vi "Read.vi"(8 "error in (no error)":errorcluster, 9 "Variant":variant, 11 "RS232 in":refnum<class "RS-xxx.lvclass">) -> (0 "error out":errorcluster, 2 "String":string, 3 "RS232 out":refnum<class "RS-xxx.lvclass">)   [LabVIEW 2013, in "Protocol Classes.lvlib" / "RS-xxx.lvclass"]
uses:
  RS-xxx.lvclass
  Protocol Parent/Methods/Read Parameter.ctl
  RS-xxx.lvclass/RS-xxx.ctl
  Data Access/Read Port Ref.vi
  Data Access/Read PortSettings.vi
  Data Access/Write Port Ref.vi
  Protocol Parent/Protocol Parent.lvclass
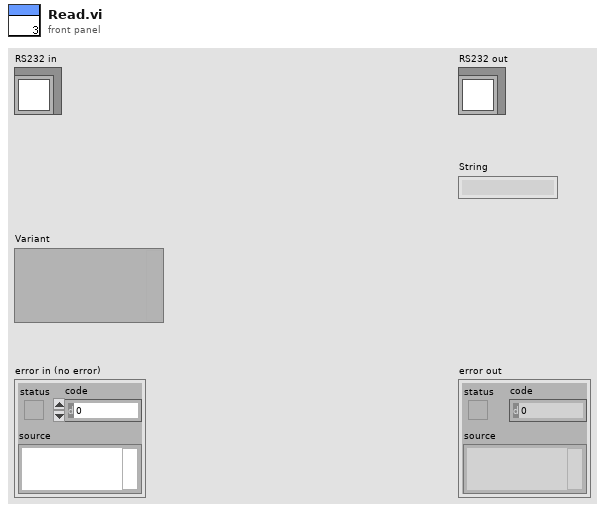
[diagram p1: front panel]
types:
  T1 = typedef "Protocol Classes.lvlib/Protocol Parent.lvclass/Read Parameter.ctl" = cluster{"Wait Type":enum16{"Byte Count", "Wait sec"}, "Wait Value":dbl}
  T2 = cluster{"Port":string, "Baud Rate":u32, "Data Bits":u16, "Parity":enum16{"None", "Odd", "Even", "Mark", "Space"}, "Stop Bits":u16, "Flow Control":u16, "XON":enum16{"NUL", "SOH", "STX", "ETX", "EOT", "ENQ", "ACK", "BEL", "BS", "HT", "LF", "VT", "FF", "CR", "SO", "SI", "DLE", "DC1", "DC2", "DC3", "DC4", "NAK", "SYN", "ETB", "CAN", "EM", "SUB", "ESC", "FS", "GS", "RS", "US", "SP", "!", "\"", "#", "$", "%", "&", "'", "(", ")", "*", "+", ",", "- (-)", ".", "/", "0", "1", "2", "3", "4", "5", "6", "7", "8", "9", ":", ";", "<", "=", ">", "?", "@", "A", "B", "C", "D", "E", "F", "G", "H", "I", "J", "K", "L", "M", "N", "O", "P", "Q", "R", "S", "T", "U", "V", "W", "X", "Y", "Z", "[", "\\", "]", "^", "_", "`", "a", "b", "c", "d", "e", "f", "g", "h", "i", "j", "k", "l", "m", "n", "o", "p", "q", "r", "s", "t", "u", "v", "w", "x", "y", "z", "{", "|", "}", "~"}, "XOFF":enum16{"NUL", "SOH", "STX", "ETX", "EOT", "ENQ", "ACK", "BEL", "BS", "HT", "LF", "VT", "FF", "CR", "SO", "SI", "DLE", "DC1", "DC2", "DC3", "DC4", "NAK", "SYN", "ETB", "CAN", "EM", "SUB", "ESC", "FS", "GS", "RS", "US", "SP", "!", "\"", "#", "$", "%", "&", "'", "(", ")", "*", "+", ",", "- (-)", ".", "/", "0", "1", "2", "3", "4", "5", "6", "7", "8", "9", ":", ";", "<", "=", ">", "?", "@", "A", "B", "C", "D", "E", "F", "G", "H", "I", "J", "K", "L", "M", "N", "O", "P", "Q", "R", "S", "T", "U", "V", "W", "X", "Y", "Z", "[", "\\", "]", "^", "_", "`", "a", "b", "c", "d", "e", "f", "g", "h", "i", "j", "k", "l", "m", "n", "o", "p", "q", "r", "s", "t", "u", "v", "w", "x", "y", "z", "{", "|", "}", "~"}, "End Read on Termination Character":bool, "End Write on Termination Character":bool, "Termination Character":u8}
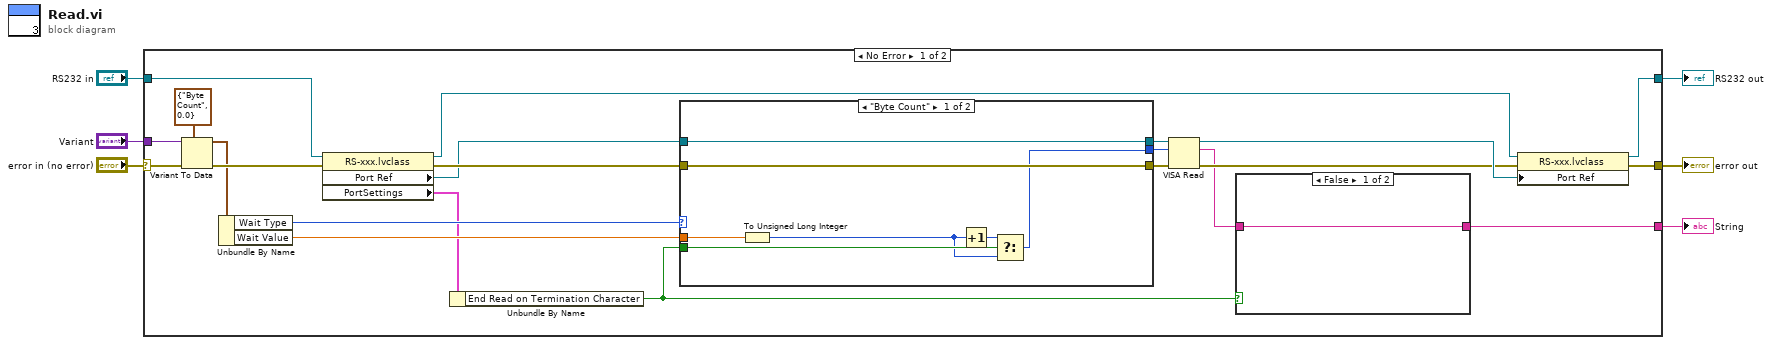
[diagram p0: block diagram]
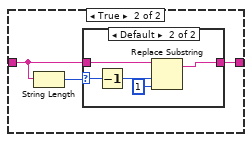
[diagram p2: hidden frame]
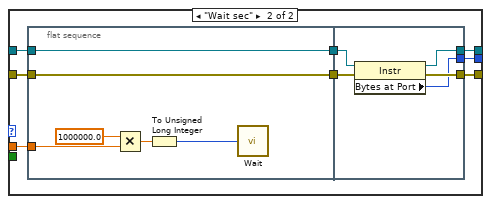
[diagram p4: hidden frame]
diagram:
  n1 = case shown="No Error" "error in (no error)" {
    selector: "error in (no error)" -> [w22 w66]
    tunnel: "RS232 in" -> [w28 w65]
    tunnel: [w25 w66] -> w2
    tunnel: [w23 w65] -> w4
    tunnel: "Variant" -> [w20 _]
    tunnel: [w8 _] -> w1
    frame No Error {
      n2 = Variant To Data(error in=w22, type=T1 {"Wait Type"=enum."Byte Count", "Wait Value"=0.0} ("Read Parameter"), Variant=w20) -> (data=w19:T1, error out=w21:errorcluster)
      n3 = Unbundle By Name(w19) -> ("Wait Type"=w13:enum16{"Byte Count", "Wait sec"}, "Wait Value"=w12:dbl)
      n4 = property class="RS-xxx.lvclass"(reference=w28, error in=w21) -> (reference out=w24:refnum<class "RS-xxx.lvclass">, error out=w18:errorcluster, "Port Ref"=w17:refnum<visa-resource-name>, "PortSettings"=w10:T2)
      n5 = Unbundle By Name(w10) -> ("End Read on Termination Character"=w7:bool)
      n6 = case shown="\"Byte Count\"" w13 {
        tunnel: w18 -> [w45 w53]
        tunnel: w17 -> [w44 w52]
        tunnel: [w45 w51] -> w16
        tunnel: [w44 w50] -> w15
        tunnel: [w40 w49] -> w14
        tunnel: w12 -> [w42 w46]
        tunnel: w7 -> [w43 _]
        frame "Byte Count" {
          n7 = To Unsigned Long Integer(number=w42) -> (unsigned 32bit integer=w39:u32)
          n8 = Increment(x=w39) -> (x+1=w41:u32)
          n9 = Select(t=w41, s=w43, f=w39) -> (s? t:f=w40:u32)
        }
        frame "Wait sec" {
          n10 = flat-sequence {
            tunnel: w52 -> [w58]
            tunnel: w53 -> [w59]
            tunnel: [w59] -> w48
            tunnel: [w58] -> w47
            tunnel: w46 -> [w55]
            tunnel: [w62] -> w51
            tunnel: [w61] -> w50
            tunnel: [w60] -> w49
            tunnel: w48 -> [w64]
            tunnel: w47 -> [w63]
            frame #0 {
              n11 = Multiply(x=1000000.0, y=w55) -> (x*y=w56:dbl)
              n12 = To Unsigned Long Integer(number=w56) -> (unsigned 32bit integer=w54:u32)
              n13 = call "Wait"("Count(uSec)"=w54) -> ()  [unwired: 1 out]
            }
            frame #1 {
              n14 = property class="Instr"(reference=w63, error in=w64) -> (reference out=w61:refnum<visa-resource-name>, error out=w62:errorcluster, "Bytes at Port"=w60:u32)
            }
          }
        }
      }
      n15 = VISA Read(VISA resource name=w15, byte count=w14, error in (no error)=w16) -> (VISA resource name out=w27:refnum<visa-resource-name>, read buffer=w9:string, error out=w26:errorcluster)  [unwired: 1 out]
      n16 = case shown="False" w7 {
        tunnel: w9 -> [w29 w31]
        tunnel: [w29 w30] -> w8
        frame False {
        }
        frame True {
          n17 = String Length(string=w31) -> (length=w32:i32)
          n18 = case shown="Default" w32 {
            selector: w32 -> [_ w38]
            tunnel: w31 -> [w33 w36]
            tunnel: [w33 w35] -> w30
            frame 0 {
            }
            frame Default {
              n19 = Decrement(x=w38) -> (x-1=w37:i32)
              n20 = Replace Substring(2:1 ("length (len. of substring)"), 3:w37, 5:w36) -> (1:w35:string)  [unwired: 1 in, 1 out]
            }
          }
        }
      }
      n21 = property class="RS-xxx.lvclass"(reference=w24, error in=w26, "Port Ref"=w27) -> (reference out=w23:refnum<class "RS-xxx.lvclass">, error out=w25:errorcluster)
    }
    frame Error {
    }
  }
  "error out" <- w2
  "RS232 out" <- w4
  "String" <- w1
